vi "draw a complex arrow.vi"(6 "number of  grid points":i32=20, 9 "to":cdb, 11 "from":cdb) -> (3 "fancy circles":cluster{dbl[], dbl[]}[](array[cluster]))   [LabVIEW 2020]
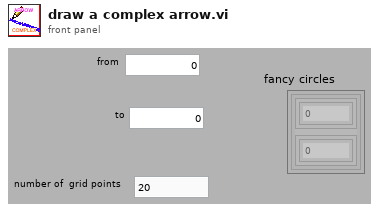
[diagram p1: front panel]
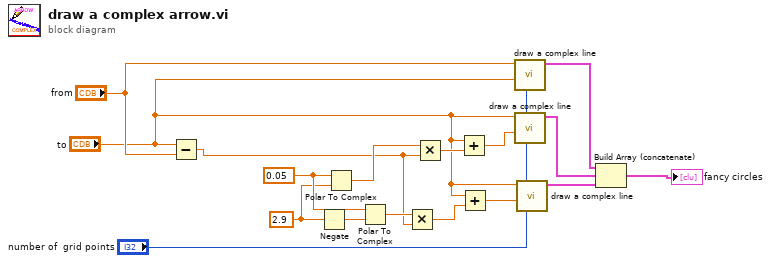
[diagram p0: block diagram]
diagram:
  w9 = 2.9 ("theta")
  w10 = 0.05 ("r")
  n1 = Subtract(x="to", y="from") -> (x-y=w6:cdb)
  n2 = Negate(x=w9) -> (-x=w8:dbl)
  n3 = Polar To Complex(1:w9, 2:w10) -> (0:w15:cdb)
  n4 = Polar To Complex(1:w8, 2:w10) -> (0:w7:cdb)
  n5 = Multiply(x=w7, y=w6) -> (x*y=w5:cdb)
  n6 = Multiply(x=w15, y=w6) -> (x*y=w17:cdb)
  n7 = Add(x="to", y=w17) -> (x+y=w12:cdb)
  n8 = Add(x="to", y=w5) -> (x+y=w4:cdb)
  n9 = call "draw a complex line.vi"("number of  grid points"="number of  grid points", "to"="to", "from"="from") -> ("array out"=w14:cluster{dbl[], dbl[]}[])  [unwired: 8 in]
  n10 = call "draw a complex line.vi"("number of  grid points"="number of  grid points", "to"=w12, "from"="to") -> ("array out"=w13:cluster{dbl[], dbl[]}[])  [unwired: 8 in]
  n11 = call "draw a complex line.vi"("to"=w4, "from"="to") -> ("array out"=w2:cluster{dbl[], dbl[]}[])  [unwired: 9 in]
  n12 = Build Array (concatenate)(w14, w13, w2) -> (→"fancy circles":cluster{dbl[], dbl[]}[])
